vi "save.vi"(8 "error in (no error)":errorcluster, 10 "Path":path, 11 "RoiCollection in":refnum<class "RoiCollection.lvclass">) -> (0 "error out":errorcluster, 3 "RoiCollection out":refnum<class "RoiCollection.lvclass">)   [LabVIEW 2010, in "RoiCollection.lvclass"]
uses:
  RoiCollection.lvclass
  RoiCollection.lvclass/RoiCollection.ctl
  RoiGeneric/RoiGeneric.lvclass
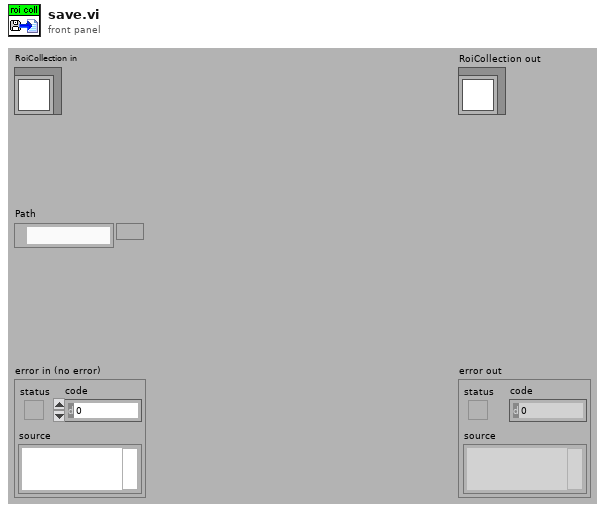
[diagram p1: front panel]
types:
  T1 = enum16{"open", "replace", "create", "open or create", "replace or create", "replace or create with confirmation"}
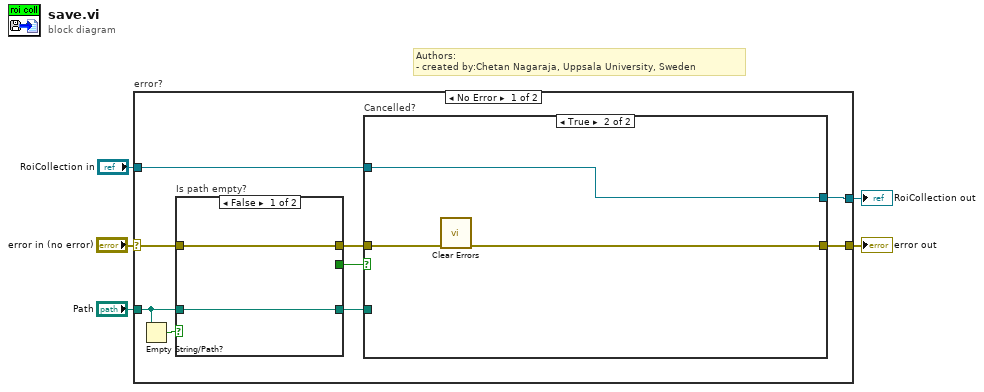
[diagram p0: block diagram]
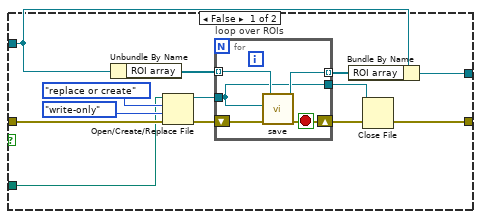
[diagram p2: hidden frame]
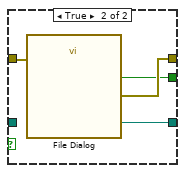
[diagram p3: hidden frame]
diagram:
  # "Authors: \n- created by:Chetan Nagaraja, Uppsala University, Sweden"
  n1 = case "error?" shown="No Error" "error in (no error)" {
    selector: "error in (no error)" -> [w11 w43]
    tunnel: [w12 w43] -> w4
    tunnel: [w13 w42] -> w2
    tunnel: "RoiCollection in" -> [w14 w42]
    tunnel: "Path" -> [w8 _]
    frame No Error {
      n2 = Empty String/Path?(string/path=w8) -> (empty?=w9:bool)
      n3 = case "Is path empty?" shown="False" w9 {
        tunnel: w11 -> [w36 w41]
        tunnel: [w36 w40] -> w10
        tunnel: [w37 w39] -> w7
        tunnel: w8 -> [w37 _]
        tunnel: [_ w38] -> w6
        frame False {
        }
        frame True {
          n4 = call "File Dialog"("error in"=w41) -> ("selected path"=w39:path, "cancelled"=w38:bool, "error out"=w40:errorcluster)  [unwired: 11 in, 1 out]
        }
      }
      n5 = case "Cancelled?" shown="True" w6 {
        tunnel: w14 -> [w21 w35]
        tunnel: [w20 w35] -> w13
        tunnel: [w18 w33] -> w12
        tunnel: w10 -> [w16 w34]
        tunnel: w7 -> [w15 _]
        frame False {
          n6 = Unbundle By Name(w21) -> ("ROI array"=w23:refnum<class "RoiGeneric.lvclass">[])
          n7 = Open/Create/Replace File(file path (use dialog)=w15, error in=w16, operation (0:open)=T1."replace or create", access (0:read/write)=enum16{"read/write", "read-only", "write-only"}."write-only") -> (refnum out=w24:refnum<file>, error out=w25:errorcluster)  [unwired: 2 in, 1 out]
          n8 = for "loop over ROIs" {
            shift-right: [w31] -> w19
            shift-left: w25 -> [w32]
            tunnel: w24 -> [w28]
            tunnel: w23 -> [w30] mode=indexing
            tunnel: [w29] -> w22 mode=indexing
            tunnel: [w28] -> w17
            stop <- w31 stop-if-true
            n9 = call-dynamic "save.vi"("error in (no error)"=w32, "file refnum in"=w28, "RoiGeneric in"=w30) -> ("error out"=w31:errorcluster, "RoiGeneric out"=w29:refnum<class "RoiGeneric.lvclass">)  [unwired: 6 in, 1 out]
          }
          n10 = Bundle By Name(cluster=w21, "ROI array"=w22) -> (w20:refnum<class "RoiCollection.lvclass">)
          n11 = Close File(2:w19, 3:w17) -> (0:w18:errorcluster)  [unwired: 1 out]
        }
        frame True {
          n12 = call <vilib>:"Clear Errors.vi"("error in (no error)"=w34) -> ("error out"=w33:errorcluster)  [unwired: 6 in]
        }
      }
    }
    frame Error {
    }
  }
  "error out" <- w4
  "RoiCollection out" <- w2
